vi "Evaluation.vi"(6 "ToEvaluate in":refnum<data-value>, 8 "error in (no error)":errorcluster, 10 "Parents G":dbl, 11 "SudukuBoard in":refnum<class "SudokuBoard.lvclass">) -> (0 "error out":errorcluster, 1 "H":dbl, 2 "G":dbl, 3 "SudukuBoard out":refnum<class "SudokuBoard.lvclass">, 4 "ToEvaluate out":refnum<data-value>)   [LabVIEW 2013, in "SudokuBoard.lvclass"]
uses:
  SudokuBoard.lvclass
  GraphNode/GraphNode.lvclass
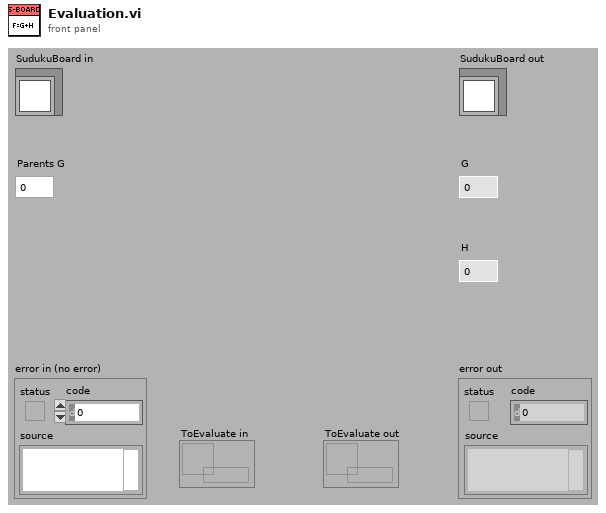
[diagram p1: front panel]
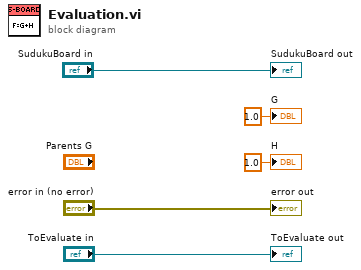
[diagram p0: block diagram]
diagram:
  "error out" <- "error in (no error)"
  "SudukuBoard out" <- "SudukuBoard in"
  "ToEvaluate out" <- "ToEvaluate in"
  "G" <- 1.0 ("G")
  "H" <- 1.0 ("H")
